vi "Check for Included Angle (scalar).vi"(6 "coerce angle":bool, 7 "angle units":T2 items=["radian in, radian out", "radian in, degree out", "degree in, degree out", "degree in, radian out"], 8 "output angle range":T1=1 items=["none", "-180 to 180 (-pi to pi)", "0 to 360 (0 to 2pi)"], 9 "end angle":dbl, 10 "start angle":dbl, 11 "angle in":dbl) -> (0 "error":i32, 2 "in range?":bool, 3 "angle out":dbl)   [LabVIEW 2020, in "NI_AAL_Angle.lvlib"]
doc: "Checks whether one or multiple input angles are within the counterclockwise range.\n\nWire data to any of the angle inputs to determine the polymorphic instance to use or manually select the instance."
uses:
  <vilib>/Analysis/NI_AAL_Angle.lvlib
  <vilib>/Analysis/coordinate.llb/Angle Units.ctl
  <vilib>/Analysis/coordinate.llb/Angle Range (Degree).ctl
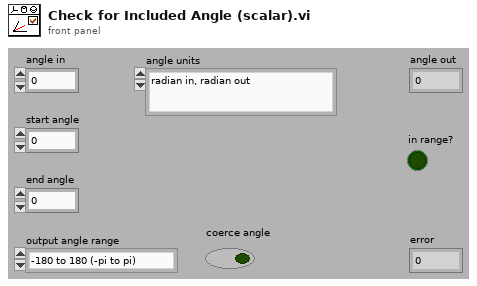
[diagram p1: front panel]
types:
  T1 = typedef "NI_AAL_Angle.lvlib/Angle Range (Degree).ctl" = u16
  T2 = typedef "NI_AAL_Angle.lvlib/Angle Units.ctl" = i32
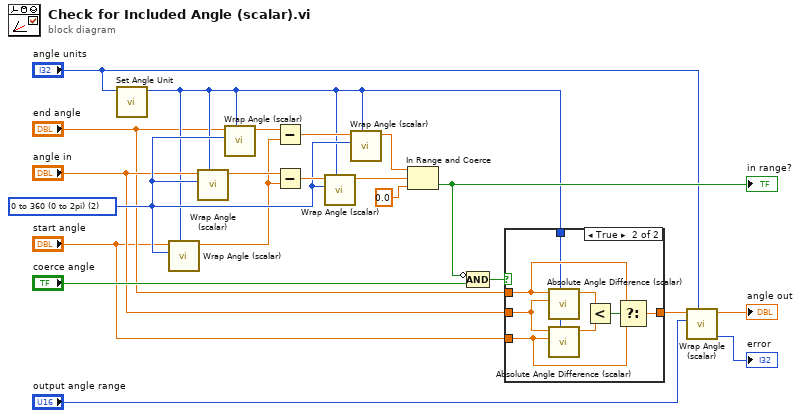
[diagram p0: block diagram]
diagram:
  w18 = T1 2 items=["none", "-180 to 180 (-pi to pi)", "0 to 360 (0 to 2pi)"] ("angle range")
  n1 = call <vilib>:"Set Angle Unit.vi"("angle units in"="angle units") -> ("angle units out"=w3:T2)  [unwired: 10 in]
  n2 = call <vilib>:"Wrap Angle (scalar).vi"("angle units"=w3, "angle range"=w18, "angle in"="start angle") -> ("angle out"=w10:dbl)  [unwired: 7 in, 1 out]
  n3 = call <vilib>:"Wrap Angle (scalar).vi"("angle units"=w3, "angle range"=w18, "angle in"="angle in") -> ("angle out"=w21:dbl)  [unwired: 7 in, 1 out]
  n4 = call <vilib>:"Wrap Angle (scalar).vi"("angle units"=w3, "angle range"=w18, "angle in"="end angle") -> ("angle out"=w11:dbl)  [unwired: 7 in, 1 out]
  n5 = Subtract(x=w11, y=w10) -> (x-y=w20:dbl)
  n6 = Subtract(x=w21, y=w10) -> (x-y=w19:dbl)
  n7 = call <vilib>:"Wrap Angle (scalar).vi"("angle units"=w3, "angle range"=w18, "angle in"=w19) -> ("angle out"=w16:dbl)  [unwired: 7 in, 1 out]
  n8 = call <vilib>:"Wrap Angle (scalar).vi"("angle units"=w3, "angle range"=w18, "angle in"=w20) -> ("angle out"=w17:dbl)  [unwired: 7 in, 1 out]
  n9 = In Range and Coerce(upper limit=w17, x=w16, lower limit=0.0) -> (In Range?=w14:bool)  [unwired: 1 out]
  "in range?" <- w14
  n10 = Compound Arithmetic op=AND(invert w14, "coerce angle") -> (w12:bool)
  n11 = case shown="True" w12 {
    tunnel: "angle in" -> [w22 w30]
    tunnel: [w22 w24] -> w8
    tunnel: "end angle" -> [_ w26]
    tunnel: "start angle" -> [_ w25]
    tunnel: w3 -> [_ w23]
    frame False {
    }
    frame True {
      n12 = call <vilib>:"Absolute Angle Difference (scalar).vi"("angle units"=w23, "angle 2"=w30, "angle 1"=w26) -> ("absolute angle difference"=w29:dbl)  [unwired: 7 in, 1 out]
      n13 = call <vilib>:"Absolute Angle Difference (scalar).vi"("angle units"=w23, "angle 2"=w25, "angle 1"=w30) -> ("absolute angle difference"=w28:dbl)  [unwired: 7 in, 1 out]
      n14 = Less?(x=w29, y=w28) -> (x < y?=w27:bool)
      n15 = Select(t=w26, s=w27, f=w25) -> (s? t:f=w24:dbl)
    }
  }
  n16 = call <vilib>:"Wrap Angle (scalar).vi"("angle units"="angle units", "angle range"="output angle range", "angle in"=w8) -> ("error"=→"error":i32, "angle out"=→"angle out":dbl)  [unwired: 7 in]
